vi "Message Queue Size.vi"(11 "Module in":refnum<class "Module.lvclass">) -> (2 "Queue Size (-1, Unlimited)":i32=-1)   [LabVIEW 2020, in "Volatus.lvlib" / "Module.lvclass"]
uses:
  Module.lvclass
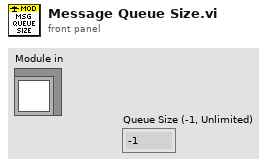
[diagram p1: front panel]
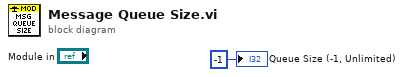
[diagram p0: block diagram]
diagram:
  "Queue Size (-1, Unlimited)" <- -1 ("Queue Size (-1)")
